vi "Create Channel Task Manual.vi"(8 "error in":errorcluster, 10 "Data":T1[](array[typedef]), 11 "NI PWM Output in":refnum<class "NI PWM Output.lvclass">) -> (0 "error out":errorcluster, 3 "NI PWM Output out":refnum<class "NI PWM Output.lvclass">)   [LabVIEW 2023, in "HardwareAbstractionLayer_LVOOP.lvlib" / "NI PWM Output.lvclass"]
doc: "This VI Analog Output Physical Channel Based DAQmx Create Channel"
uses:
  NI PWM Output.lvclass
  GUI/Actor/Diagnostic/Instruments UI/PWM Output/Control/PWM Output.ctl
  NI PWM Output.lvclass/NI PWM Output.ctl
  <vilib>/DAQmx/create/channels.llb/DAQmx Create Channel (CO-Pulse Generation-Frequency).vi
  <vilib>/DAQmx/configure/timing.llb/DAQmx Timing (Implicit).vi
  <resource>/objmgr/daqmx.rc
  GUI/Actor/Diagnostic/Diagnostic.lvlib
panel:
  out "CO Pulse Duty Cycle":dbl[](array[numeric])
  out "CO Pulse Frequency":dbl[](array[numeric])
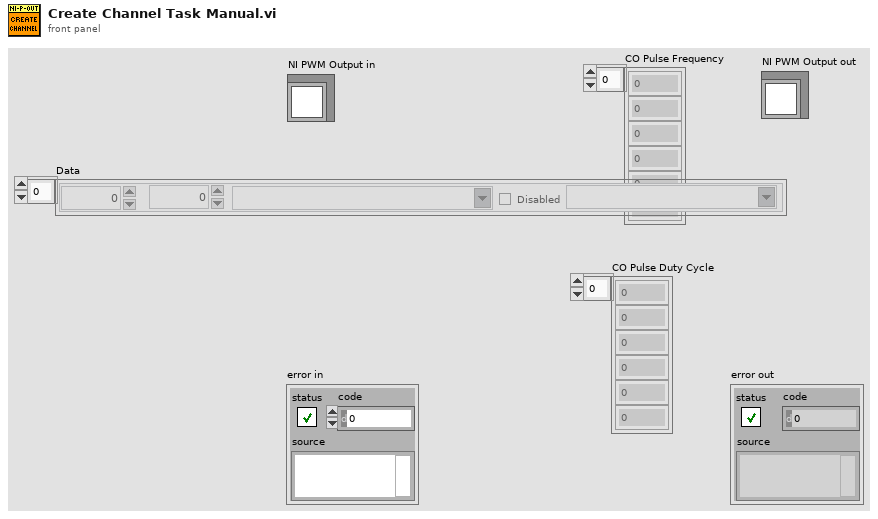
[diagram p1: front panel]
types:
  T1 = typedef "GUI.lvlib/Diagnostic.lvlib/PWM Output.ctl" = cluster{"Frequency":dbl, "Duty Cycles":dbl, "Terminal":tag, "Enable":bool, "Physical Channel":tag}
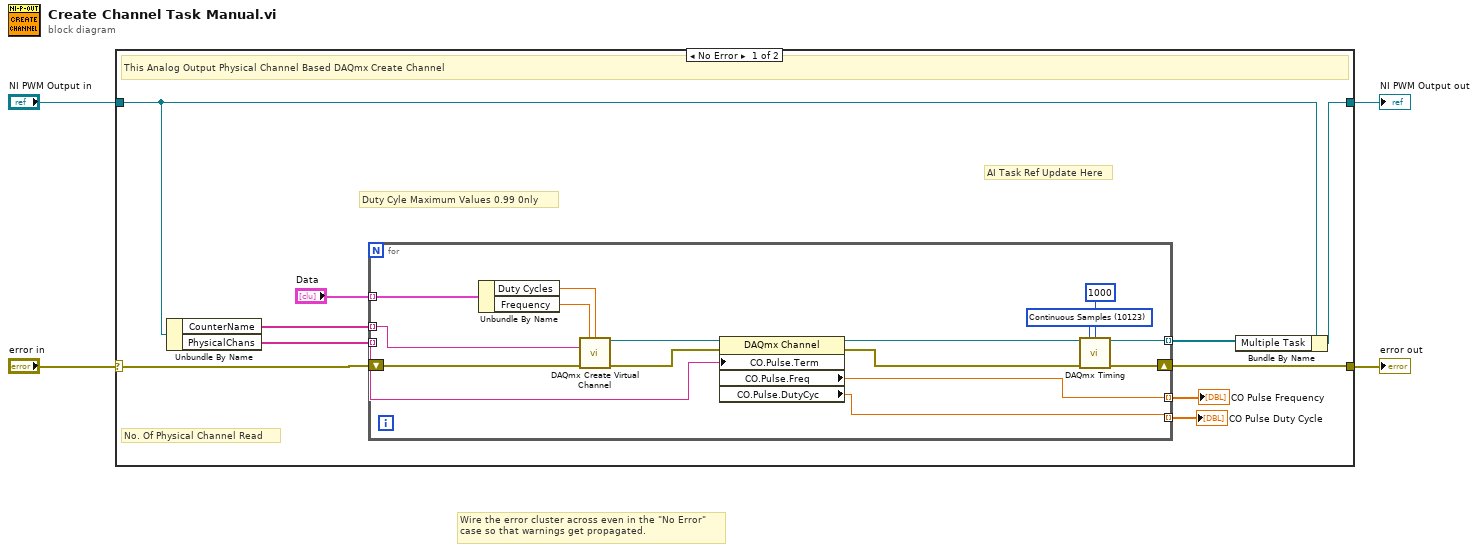
[diagram p0: block diagram]
diagram:
  # "Wire the error cluster across even in the \"No Error\"\ncase so that warnings get propagated."
  n1 = case shown="No Error" "error in" {
    selector: "error in" -> [w6 w32]
    tunnel: [w11 w32] -> w3
    tunnel: [w13 w31] -> w1
    tunnel: "NI PWM Output in" -> [w12 w31]
    frame No Error {
      # "Duty Cyle Maximum Values 0.99 0nly"
      # "AI Task Ref Update Here"
      # "No. Of Physical Channel Read"
      # "This Analog Output Physical Channel Based DAQmx Create Channel"
      n2 = Unbundle By Name(w12) -> ("CounterName"=w7:tag[], "PhysicalChans"=w10:tag[])
      n3 = for {
        tunnel: [w29] -> w14 mode=indexing
        tunnel: w10 -> [w26] mode=indexing
        tunnel: [w25] -> w9 mode=indexing
        tunnel: [w24] -> w8 mode=indexing
        tunnel: w7 -> [w23] mode=indexing
        tunnel: "Data" -> [w20] mode=indexing
        shift-right: [w28] -> w11
        shift-left: w6 -> [w21]
        w30 = 10123 items=["Finite Samples"=10178, "Continuous Samples"=10123, "Hardware Timed Single Point"=12522] ("sample mode")
        n4 = Unbundle By Name(w20) -> ("Duty Cycles"=w17:dbl, "Frequency"=w16:dbl)
        n5 = call-poly <vilib>:"DAQmx Create Virtual Channel.vi"("frequency"=w16, "duty cycle"=w17, "counter"=w23, "error in"=w21) -> ("task out"=w19:refnum<k21>, "error out"=w18:errorcluster)  [unwired: 10 in]
        n6 = property class="DAQmx Channel"(reference=w19, error in=w18, "CO.Pulse.Term"=w26) -> (reference out=w22:refnum<k21>, error out=w27:errorcluster, "CO.Pulse.Freq"=w25:dbl, "CO.Pulse.DutyCyc"=w24:dbl)
        n7 = call-poly <vilib>:"DAQmx Timing.vi"("task/channels in"=w22, "sample mode"=w30, "samples per channel"=1000, "error in"=w27) -> ("task out"=w29:refnum<k21>, "error out"=w28:errorcluster)  [unwired: 10 in]
      }
      "CO Pulse Frequency" <- w9
      "CO Pulse Duty Cycle" <- w8
      n8 = Bundle By Name(cluster=w12, "Multiple Task"=w14) -> (w13:refnum<class "NI PWM Output.lvclass">)
    }
    frame Error {
    }
  }
  "error out" <- w3
  "NI PWM Output out" <- w1
